vi "reshape array.vi"(8 "error in (no error)":errorcluster, 10 "array":u8[](array[numeric]), 11 "Thorcam in":refnum<class "Thorcam.lvclass">) -> (0 "error out":errorcluster, 2 "image array out":u8[][](array[numeric]), 3 "Thorcam out":refnum<class "Thorcam.lvclass">)   [LabVIEW 2012, in "Thorcam.lvclass"]
uses:
  Thorcam.lvclass
  Thorcam.lvclass/Thorcam.ctl
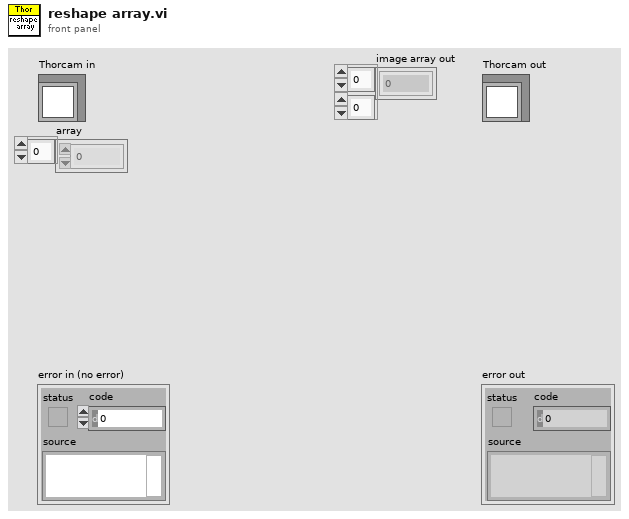
[diagram p1: front panel]
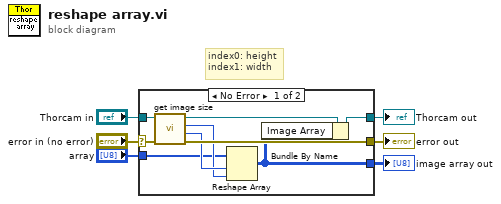
[diagram p0: block diagram]
diagram:
  # "index0: height\nindex1: width"
  n1 = case shown="No Error" "error in (no error)" {
    selector: "error in (no error)" -> [w15 w17]
    tunnel: [w14 w17] -> w5
    tunnel: [w11 w16] -> w3
    tunnel: "Thorcam in" -> [w13 w16]
    tunnel: "array" -> [w8 _]
    tunnel: [w7 _] -> w1
    frame No Error {
      n2 = call-dynamic "get image size.vi"("error in (no error)"=w15, "Thorcam in"=w13) -> ("error out"=w14:errorcluster, "Height"=w10:i32, "Width"=w9:i32, "Thorcam out"=w12:refnum<class "Thorcam.lvclass">)  [unwired: 6 in]
      n3 = Reshape Array(w8, w10, w9) -> (w7:u8[][])
      n4 = Bundle By Name(cluster=w12, "Image Array"=w7) -> (w11:refnum<class "Thorcam.lvclass">)
    }
    frame Error {
    }
  }
  "error out" <- w5
  "Thorcam out" <- w3
  "image array out" <- w1
